vi "Build Evaluation String.vi"(6 "VI Path":path, 7 "Assert Scripting Configuration":T1={"Assert Name"="", "Comment"="", "Numeric Operation"="", "Type"=enum."Double Float", "String Operation"="", "DBL Comparison Value 1"=0.0, "DBL Comparison Value 2"=0.0, "I32 Comparison Value 1"=0, "I32 Comparison Value 2"=0, "Creator"="", "Creation Timestamp"=timestamp(0 s since 1904-01-01), "String Comparison Value"="", "Description"="", "Default Failure Action"=enum."None", "Boolean Comparison Value"=FALSE, "I8 Comparison Value 1"=0, "I8 Comparison Value 2"=0, "I16 Comparison Value 1"=0, "I16 Comparison Value 2"=0, "I64 Comparison Value 1"=0, "I64 Comparison Value 2"=0, "U8 Comparison Value 1"=0, "U8 Comparison Value 2"=0, "U16 Comparison Value 1"=0, "U16 Comparison Value 2"=0, "U32 Comparison Value 1"=0, "U32 Comparison Value 2"=0, "U64 Comparison Value 1"=0, "U64 Comparison Value 2"=0, "EXT Comparison Value 1"=0.0, "EXT Comparison Value 2"=0.0, "SGL Comparison Value 1"=0.0, "SGL Comparison Value 2"=0.0}, 8 "error in (no error)":errorcluster) -> (0 "error out":errorcluster, 2 "Evaluation String":string)   [LabVIEW 2016]
doc: "Builds up an evaluation string based on the input parameters specified and applies it to the new assert test vi."
uses:
  Assert Scripting Configuration.ctl
  <vilib>/Utility/Data Type/Type Definitions/Data Type.ctl
  <vilib>/Utility/error.llb/Error Cluster From Error Code.vi
  <vilib>/ErrorRing/Error Ring.xnode
  <vilib>/Utility/Data Type/NI_Data Type.lvlib
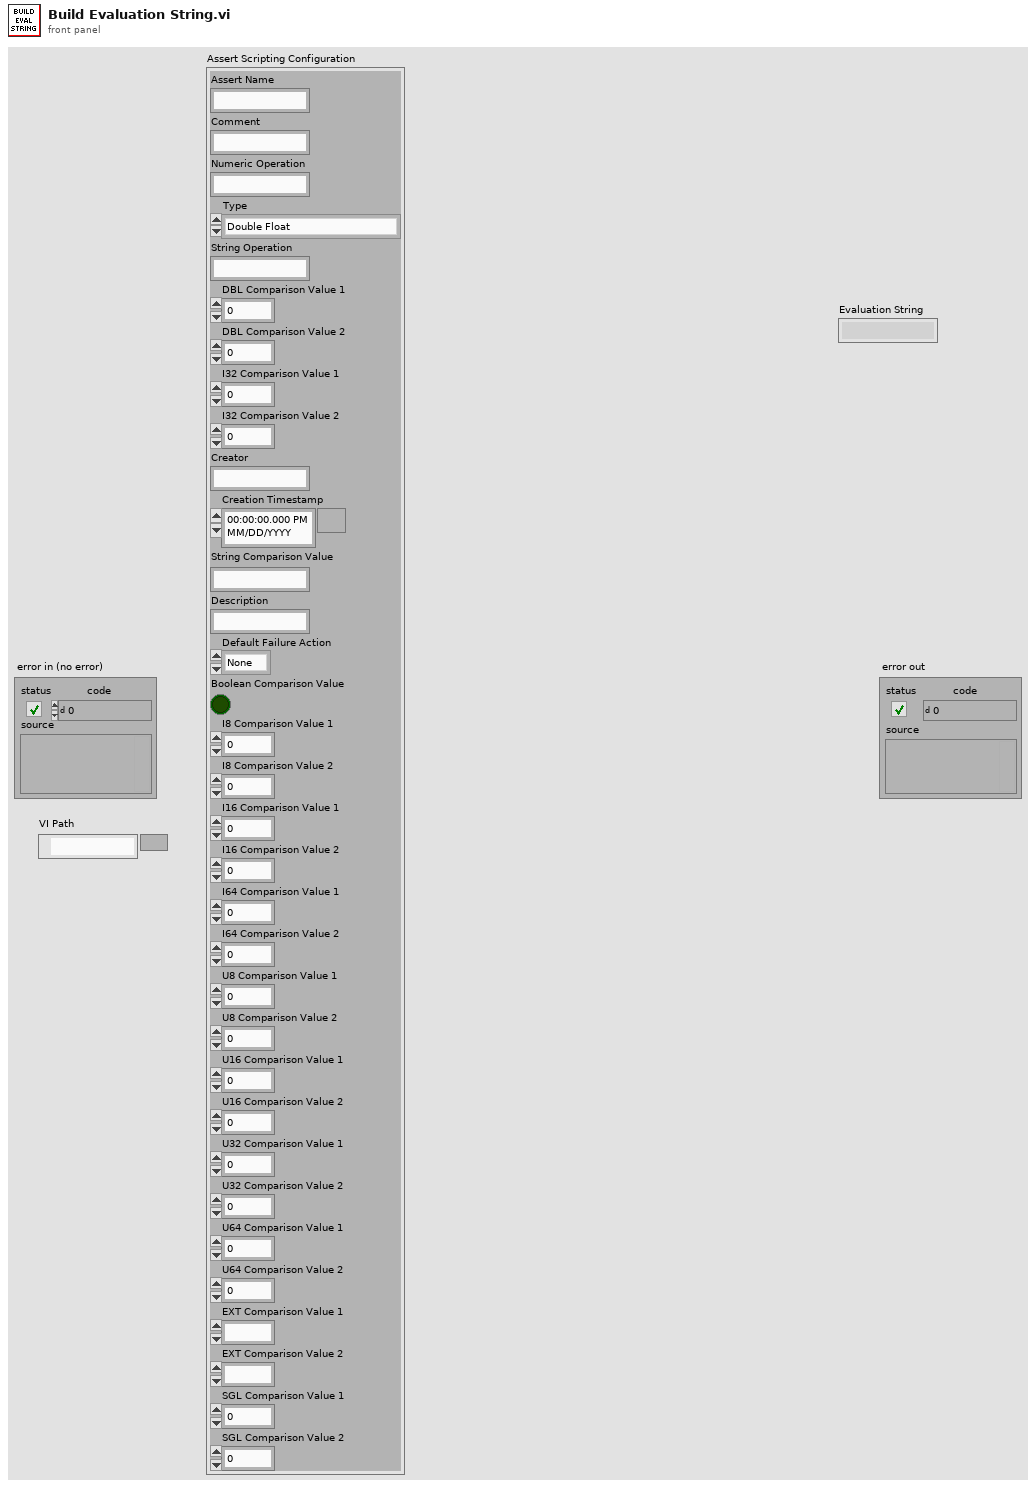
[diagram p1: front panel]
types:
  T1 = typedef "Assert Scripting Configuration.ctl" = cluster{"Assert Name":string, "Comment":string, "Numeric Operation":string, "Type":T2, "String Operation":string, "DBL Comparison Value 1":dbl, "DBL Comparison Value 2":dbl, "I32 Comparison Value 1":i32, "I32 Comparison Value 2":i32, "Creator":string, "Creation Timestamp":timestamp, "String Comparison Value":string, "Description":string, "Default Failure Action":enum16{"None", "Log To File", "Pause Execution", "Abort Execution"}, "Boolean Comparison Value":bool, "I8 Comparison Value 1":i8, "I8 Comparison Value 2":i8, "I16 Comparison Value 1":i16, "I16 Comparison Value 2":i16, "I64 Comparison Value 1":i64, "I64 Comparison Value 2":i64, "U8 Comparison Value 1":u8, "U8 Comparison Value 2":u8, "U16 Comparison Value 1":u16, "U16 Comparison Value 2":u16, "U32 Comparison Value 1":u32, "U32 Comparison Value 2":u32, "U64 Comparison Value 1":u64, "U64 Comparison Value 2":u64, "EXT Comparison Value 1":ext, "EXT Comparison Value 2":ext, "SGL Comparison Value 1":sgl, "SGL Comparison Value 2":sgl}
  T2 = typedef "NI_Data Type.lvlib/Data Type.ctl" = enum8{"Invalid Type", "Void", "I8", "I16", "I32", "I64", "U8", "U16", "U32", "U64", "Single Float", "Double Float", "Extended Float", "Single Complex", "Double Complex", "Extended Complex", "Enum U8", "Enum U16", "Enum U32", "Enum U64", "Single Float With Unit", "Double Float With Unit", "Extended Float With Unit", "Single Complex with Unit", "Double Complex with Unit", "Extended Complex with Unit", "Boolean", "String", "Path", "Picture", "Tag", "Array", "Cluster", "Variant", "LV Variant", "Waveform", "Timestamp", "Digital Waveform", "Digital Data", "ExpressData", "Refnum", "External Data", "VI", "Poly VI", "LabVIEW Class Instance", "Fixed Point"}
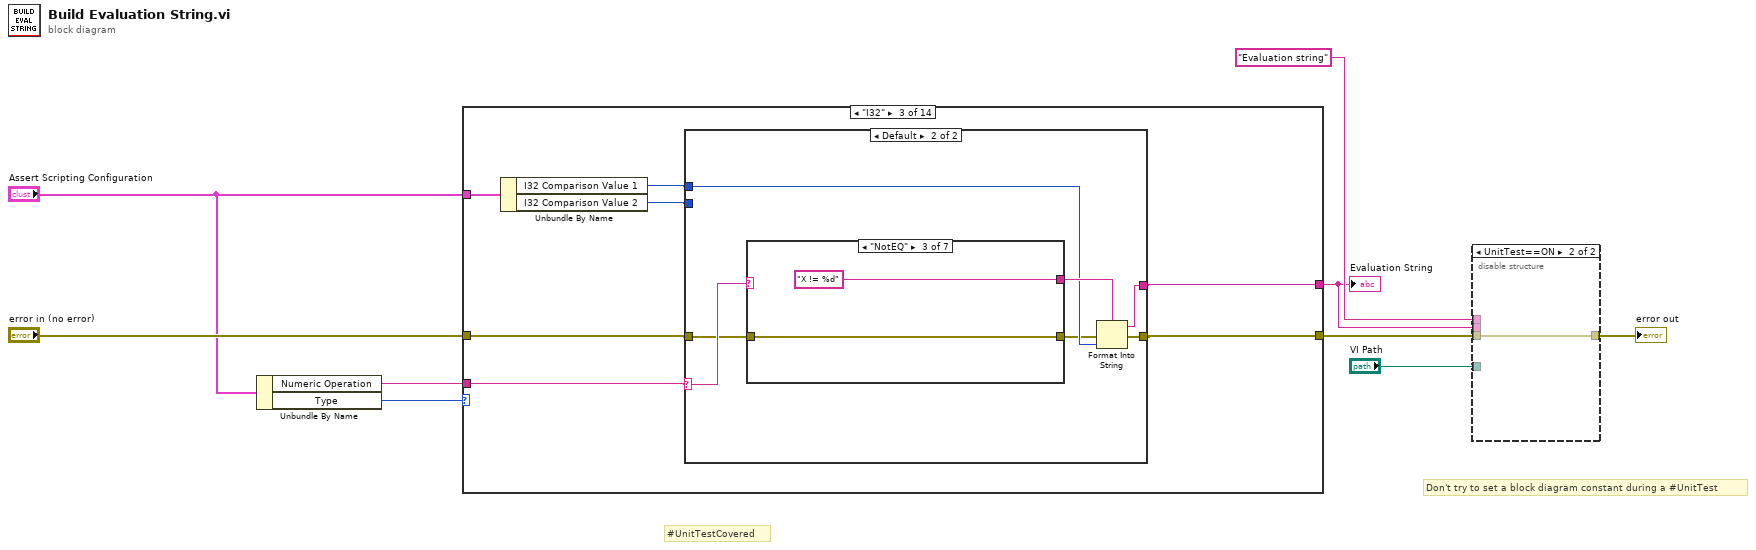
[diagram p0: block diagram]
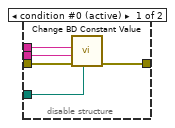
[diagram p2: hidden frame]
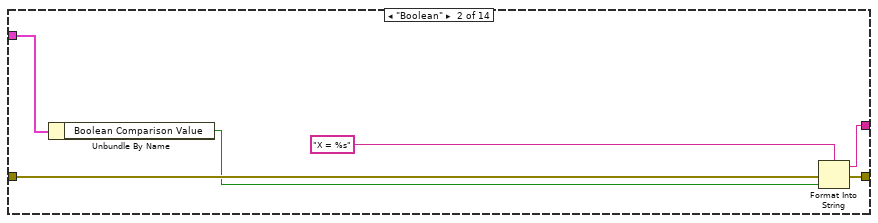
[diagram p4: hidden frame]
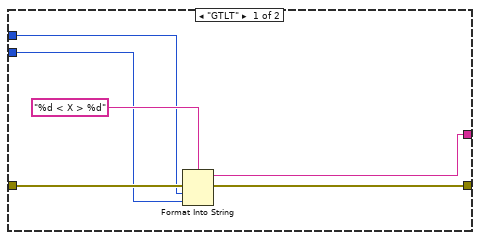
[diagram p5: hidden frame]
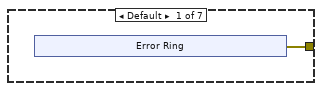
[diagram p6: hidden frame]
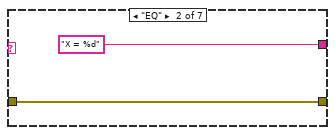
[diagram p7: hidden frame]
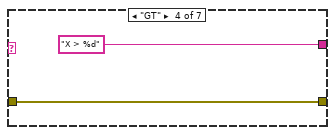
[diagram p8: hidden frame]
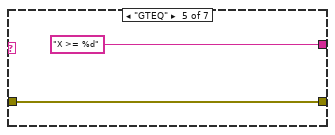
[diagram p9: hidden frame]
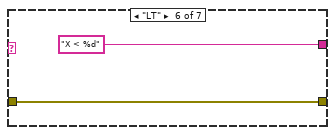
[diagram p10: hidden frame]
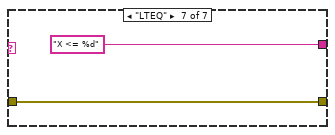
[diagram p11: hidden frame]
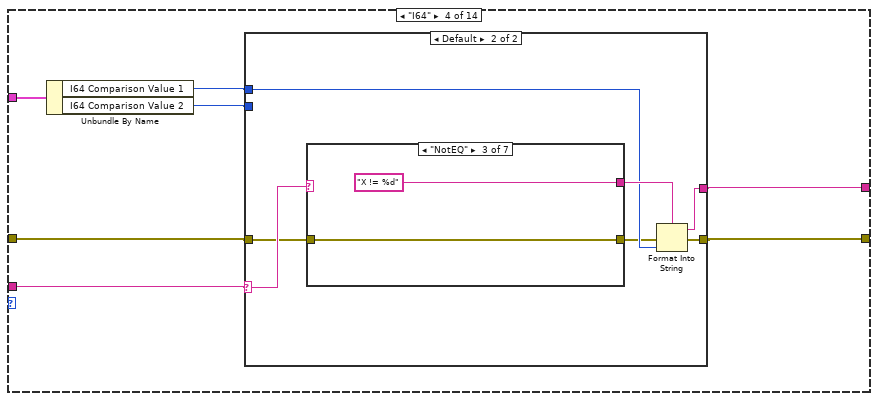
[diagram p12: hidden frame]
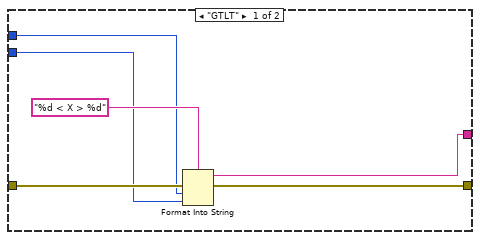
[diagram p13: hidden frame]
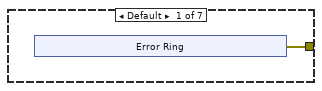
[diagram p14: hidden frame]
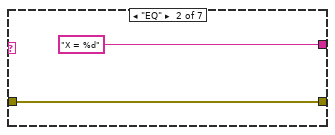
[diagram p15: hidden frame]
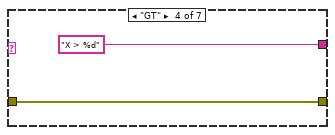
[diagram p16: hidden frame]
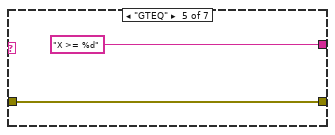
[diagram p17: hidden frame]
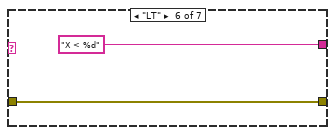
[diagram p18: hidden frame]
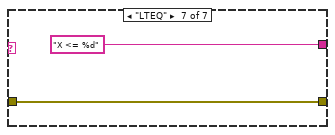
[diagram p19: hidden frame]
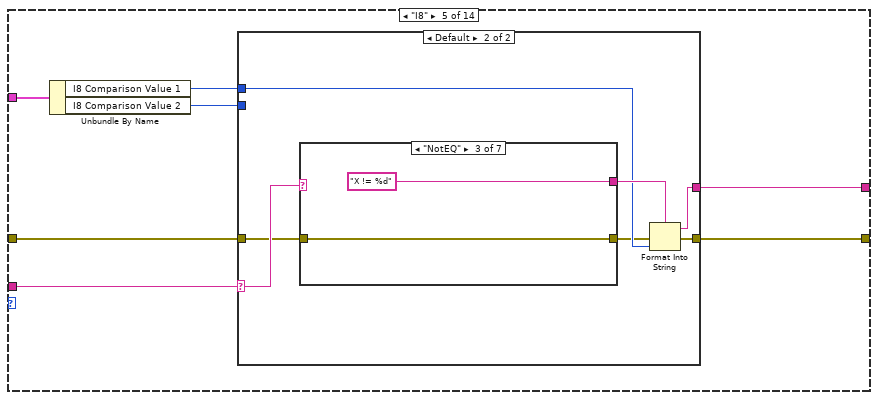
[diagram p20: hidden frame]
diagram:
  # "#UnitTestCovered"
  # "Don't try to set a block diagram constant during a #UnitTest"
  n1 = Unbundle By Name("Assert Scripting Configuration") -> ("Numeric Operation"=w7:string, "Type"=w8:T2)
  n2 = case shown="\"I32\"" w8 {
    tunnel: w7 -> [_ _ w22 w60 w98 w136 w174 w209 w250 w286 w323 w364 w403 _]
    tunnel: [_ w15 w18 w56 w94 w132 w170 w207 w246 w283 w321 w360 w402 w438] -> w5
    tunnel: "error in (no error)" -> [w10 w14 w21 w59 w97 w135 w173 w210 w249 w285 w324 w363 w401 w441]
    tunnel: [w10 w13 w17 w55 w93 w131 w169 w208 w245 w284 w322 w359 w400 w440] -> w4
    tunnel: "Assert Scripting Configuration" -> [_ w12 w23 w61 w99 w137 w175 w213 w251 w289 w327 w365 w399 w437]
    frame Default {
    }
    frame "Boolean" {
      n3 = Unbundle By Name(w12) -> ("Boolean Comparison Value"=w11:bool)
      n4 = Format Into String(format string="X = %s", error in=w14, w11) -> (resulting string=w15:string, error out=w13:errorcluster)  [unwired: 1 in]
    }
    frame "I32" {
      n5 = Unbundle By Name(w23) -> ("I32 Comparison Value 1"=w19:i32, "I32 Comparison Value 2"=w20:i32)
      n6 = case shown="Default" w22 {
        selector: w22 -> [_ w36]
        tunnel: [w28 w34] -> w18
        tunnel: w21 -> [w27 w31]
        tunnel: [w26 w33] -> w17
        tunnel: w19 -> [w25 w32]
        tunnel: w20 -> [w24 _]
        frame "GTLT" {
          n7 = Format Into String(format string="%d < X > %d", error in=w27, w25, w24) -> (resulting string=w28:string, error out=w26:errorcluster)  [unwired: 1 in]
        }
        frame Default {
          n8 = case shown="\"NotEQ\"" w36 {
            tunnel: [_ "X = %d" "X != %d" "X > %d" "X >= %d" "X < %d" "X <= %d"] -> w35
            tunnel: w31 -> [_ w43 w45 w47 w49 w51 w53]
            tunnel: [w37 w43 w45 w47 w49 w51 w53] -> w30
            frame Default {
              n9 = xnode "Error Ring"() -> ("error out"=w37:errorcluster)
            }
            frame "EQ" {
            }
            frame "NotEQ" {
            }
            frame "GT" {
            }
            frame "GTEQ" {
            }
            frame "LT" {
            }
            frame "LTEQ" {
            }
          }
          n10 = Format Into String(format string=w35, error in=w30, w32) -> (resulting string=w34:string, error out=w33:errorcluster)  [unwired: 1 in]
        }
      }
    }
    frame "I64" {
      n11 = Unbundle By Name(w61) -> ("I64 Comparison Value 1"=w57:i64, "I64 Comparison Value 2"=w58:i64)
      n12 = case shown="Default" w60 {
        selector: w60 -> [_ w74]
        tunnel: [w66 w72] -> w56
        tunnel: w59 -> [w65 w69]
        tunnel: [w64 w71] -> w55
        tunnel: w57 -> [w63 w70]
        tunnel: w58 -> [w62 _]
        frame "GTLT" {
          n13 = Format Into String(format string="%d < X > %d", error in=w65, w63, w62) -> (resulting string=w66:string, error out=w64:errorcluster)  [unwired: 1 in]
        }
        frame Default {
          n14 = case shown="\"NotEQ\"" w74 {
            tunnel: [_ "X = %d" "X != %d" "X > %d" "X >= %d" "X < %d" "X <= %d"] -> w73
            tunnel: w69 -> [_ w81 w83 w85 w87 w89 w91]
            tunnel: [w75 w81 w83 w85 w87 w89 w91] -> w68
            frame Default {
              n15 = xnode "Error Ring"() -> ("error out"=w75:errorcluster)
            }
            frame "EQ" {
            }
            frame "NotEQ" {
            }
            frame "GT" {
            }
            frame "GTEQ" {
            }
            frame "LT" {
            }
            frame "LTEQ" {
            }
          }
          n16 = Format Into String(format string=w73, error in=w68, w70) -> (resulting string=w72:string, error out=w71:errorcluster)  [unwired: 1 in]
        }
      }
    }
    frame "I8" {
      n17 = Unbundle By Name(w99) -> ("I8 Comparison Value 1"=w95:i8, "I8 Comparison Value 2"=w96:i8)
      n18 = case shown="Default" w98 {
        selector: w98 -> [_ w112]
        tunnel: [w104 w110] -> w94
        tunnel: w97 -> [w103 w107]
        tunnel: [w102 w109] -> w93
        tunnel: w95 -> [w101 w108]
        tunnel: w96 -> [w100 _]
        frame "GTLT" {
          n19 = Format Into String(format string="%d < X > %d", error in=w103, w101, w100) -> (resulting string=w104:string, error out=w102:errorcluster)  [unwired: 1 in]
        }
        frame Default {
          n20 = case shown="\"NotEQ\"" w112 {
            tunnel: [_ "X = %d" "X != %d" "X > %d" "X >= %d" "X < %d" "X <= %d"] -> w111
            tunnel: w107 -> [_ w119 w121 w123 w125 w127 w129]
            tunnel: [w113 w119 w121 w123 w125 w127 w129] -> w106
            frame Default {
              n21 = xnode "Error Ring"() -> ("error out"=w113:errorcluster)
            }
            frame "EQ" {
            }
            frame "NotEQ" {
            }
            frame "GT" {
            }
            frame "GTEQ" {
            }
            frame "LT" {
            }
            frame "LTEQ" {
            }
          }
          n22 = Format Into String(format string=w111, error in=w106, w108) -> (resulting string=w110:string, error out=w109:errorcluster)  [unwired: 1 in]
        }
      }
    }
    frame "I16" {
      n23 = Unbundle By Name(w137) -> ("I16 Comparison Value 1"=w133:i16, "I16 Comparison Value 2"=w134:i16)
      n24 = case shown="Default" w136 {
        selector: w136 -> [_ w150]
        tunnel: [w142 w148] -> w132
        tunnel: w135 -> [w141 w145]
        tunnel: [w140 w147] -> w131
        tunnel: w133 -> [w139 w146]
        tunnel: w134 -> [w138 _]
        frame "GTLT" {
          n25 = Format Into String(format string="%d < X > %d", error in=w141, w139, w138) -> (resulting string=w142:string, error out=w140:errorcluster)  [unwired: 1 in]
        }
        frame Default {
          n26 = case shown="\"NotEQ\"" w150 {
            tunnel: [_ "X = %d" "X != %d" "X > %d" "X >= %d" "X < %d" "X <= %d"] -> w149
            tunnel: w145 -> [_ w157 w159 w161 w163 w165 w167]
            tunnel: [w151 w157 w159 w161 w163 w165 w167] -> w144
            frame Default {
              n27 = xnode "Error Ring"() -> ("error out"=w151:errorcluster)
            }
            frame "EQ" {
            }
            frame "NotEQ" {
            }
            frame "GT" {
            }
            frame "GTEQ" {
            }
            frame "LT" {
            }
            frame "LTEQ" {
            }
          }
          n28 = Format Into String(format string=w149, error in=w144, w146) -> (resulting string=w148:string, error out=w147:errorcluster)  [unwired: 1 in]
        }
      }
    }
    frame "U8" {
      n29 = Unbundle By Name(w175) -> ("U8 Comparison Value 1"=w171:u8, "U8 Comparison Value 2"=w172:u8)
      n30 = case shown="Default" w174 {
        selector: w174 -> [_ w188]
        tunnel: [w180 w186] -> w170
        tunnel: w173 -> [w179 w183]
        tunnel: [w178 w185] -> w169
        tunnel: w171 -> [w177 w184]
        tunnel: w172 -> [w176 _]
        frame "GTLT" {
          n31 = Format Into String(format string="%d < X > %d", error in=w179, w177, w176) -> (resulting string=w180:string, error out=w178:errorcluster)  [unwired: 1 in]
        }
        frame Default {
          n32 = case shown="\"NotEQ\"" w188 {
            tunnel: [_ "X = %d" "X != %d" "X > %d" "X >= %d" "X < %d" "X <= %d"] -> w187
            tunnel: w183 -> [_ w195 w197 w199 w201 w203 w205]
            tunnel: [w189 w195 w197 w199 w201 w203 w205] -> w182
            frame Default {
              n33 = xnode "Error Ring"() -> ("error out"=w189:errorcluster)
            }
            frame "EQ" {
            }
            frame "NotEQ" {
            }
            frame "GT" {
            }
            frame "GTEQ" {
            }
            frame "LT" {
            }
            frame "LTEQ" {
            }
          }
          n34 = Format Into String(format string=w187, error in=w182, w184) -> (resulting string=w186:string, error out=w185:errorcluster)  [unwired: 1 in]
        }
      }
    }
    frame "U16" {
      n35 = Unbundle By Name(w213) -> ("U16 Comparison Value 1"=w212:u16, "U16 Comparison Value 2"=w211:u16)
      n36 = case shown="Default" w209 {
        selector: w209 -> [_ w226]
        tunnel: [w218 w224] -> w207
        tunnel: w210 -> [w217 w221]
        tunnel: [w216 w223] -> w208
        tunnel: w212 -> [w215 w222]
        tunnel: w211 -> [w214 _]
        frame "GTLT" {
          n37 = Format Into String(format string="%d < X > %d", error in=w217, w215, w214) -> (resulting string=w218:string, error out=w216:errorcluster)  [unwired: 1 in]
        }
        frame Default {
          n38 = case shown="\"NotEQ\"" w226 {
            tunnel: [_ "X = %d" "X != %d" "X > %d" "X >= %d" "X < %d" "X <= %d"] -> w225
            tunnel: w221 -> [_ w233 w235 w237 w239 w241 w243]
            tunnel: [w227 w233 w235 w237 w239 w241 w243] -> w220
            frame Default {
              n39 = xnode "Error Ring"() -> ("error out"=w227:errorcluster)
            }
            frame "EQ" {
            }
            frame "NotEQ" {
            }
            frame "GT" {
            }
            frame "GTEQ" {
            }
            frame "LT" {
            }
            frame "LTEQ" {
            }
          }
          n40 = Format Into String(format string=w225, error in=w220, w222) -> (resulting string=w224:string, error out=w223:errorcluster)  [unwired: 1 in]
        }
      }
    }
    frame "U32" {
      n41 = Unbundle By Name(w251) -> ("U32 Comparison Value 1"=w247:u32, "U32 Comparison Value 2"=w248:u32)
      n42 = case shown="Default" w250 {
        selector: w250 -> [_ w264]
        tunnel: [w256 w262] -> w246
        tunnel: w249 -> [w255 w259]
        tunnel: [w254 w261] -> w245
        tunnel: w247 -> [w253 w260]
        tunnel: w248 -> [w252 _]
        frame "GTLT" {
          n43 = Format Into String(format string="%d < X > %d", error in=w255, w253, w252) -> (resulting string=w256:string, error out=w254:errorcluster)  [unwired: 1 in]
        }
        frame Default {
          n44 = case shown="\"NotEQ\"" w264 {
            tunnel: [_ "X = %d" "X != %d" "X > %d" "X >= %d" "X < %d" "X <= %d"] -> w263
            tunnel: w259 -> [_ w271 w273 w275 w277 w279 w281]
            tunnel: [w265 w271 w273 w275 w277 w279 w281] -> w258
            frame Default {
              n45 = xnode "Error Ring"() -> ("error out"=w265:errorcluster)
            }
            frame "EQ" {
            }
            frame "NotEQ" {
            }
            frame "GT" {
            }
            frame "GTEQ" {
            }
            frame "LT" {
            }
            frame "LTEQ" {
            }
          }
          n46 = Format Into String(format string=w263, error in=w258, w260) -> (resulting string=w262:string, error out=w261:errorcluster)  [unwired: 1 in]
        }
      }
    }
    frame "U64" {
      n47 = Unbundle By Name(w289) -> ("U64 Comparison Value 1"=w288:u64, "U64 Comparison Value 2"=w287:u64)
      n48 = case shown="Default" w286 {
        selector: w286 -> [_ w302]
        tunnel: [w294 w300] -> w283
        tunnel: w285 -> [w293 w297]
        tunnel: [w292 w299] -> w284
        tunnel: w288 -> [w291 w298]
        tunnel: w287 -> [w290 _]
        frame "GTLT" {
          n49 = Format Into String(format string="%d < X > %d", error in=w293, w291, w290) -> (resulting string=w294:string, error out=w292:errorcluster)  [unwired: 1 in]
        }
        frame Default {
          n50 = case shown="\"NotEQ\"" w302 {
            tunnel: [_ "X = %d" "X != %d" "X > %d" "X >= %d" "X < %d" "X <= %d"] -> w301
            tunnel: w297 -> [_ w309 w311 w313 w315 w317 w319]
            tunnel: [w303 w309 w311 w313 w315 w317 w319] -> w296
            frame Default {
              n51 = xnode "Error Ring"() -> ("error out"=w303:errorcluster)
            }
            frame "EQ" {
            }
            frame "NotEQ" {
            }
            frame "GT" {
            }
            frame "GTEQ" {
            }
            frame "LT" {
            }
            frame "LTEQ" {
            }
          }
          n52 = Format Into String(format string=w301, error in=w296, w298) -> (resulting string=w300:string, error out=w299:errorcluster)  [unwired: 1 in]
        }
      }
    }
    frame "Double Float" {
      n53 = Unbundle By Name(w327) -> ("DBL Comparison Value 1"=w325:dbl, "DBL Comparison Value 2"=w326:dbl)
      n54 = case shown="\"GTLT\"" w323 {
        selector: w323 -> [_ w340]
        tunnel: [w332 w338] -> w321
        tunnel: w324 -> [w331 w335]
        tunnel: [w330 w337] -> w322
        tunnel: w325 -> [w329 w336]
        tunnel: w326 -> [w328 _]
        frame "GTLT" {
          n55 = Format Into String(format string="%f < X > %f", error in=w331, w329, w328) -> (resulting string=w332:string, error out=w330:errorcluster)  [unwired: 1 in]
        }
        frame Default {
          n56 = case shown="\"EQ\"" w340 {
            tunnel: [_ "X = %f" "X != %f" "X > %f" "X >= %f" "X < %f" "X <= %f"] -> w339
            tunnel: w335 -> [_ w347 w349 w351 w353 w355 w357]
            tunnel: [w341 w347 w349 w351 w353 w355 w357] -> w334
            frame Default {
              n57 = xnode "Error Ring"() -> ("error out"=w341:errorcluster)
            }
            frame "EQ" {
            }
            frame "NotEQ" {
            }
            frame "GT" {
            }
            frame "GTEQ" {
            }
            frame "LT" {
            }
            frame "LTEQ" {
            }
          }
          n58 = Format Into String(format string=w339, error in=w334, w336) -> (resulting string=w338:string, error out=w337:errorcluster)  [unwired: 1 in]
        }
      }
    }
    frame "Extended Float" {
      n59 = Unbundle By Name(w365) -> ("EXT Comparison Value 1"=w361:ext, "EXT Comparison Value 2"=w362:ext)
      n60 = case shown="\"GTLT\"" w364 {
        selector: w364 -> [_ w378]
        tunnel: [w370 w376] -> w360
        tunnel: w363 -> [w369 w373]
        tunnel: [w368 w375] -> w359
        tunnel: w361 -> [w367 w374]
        tunnel: w362 -> [w366 _]
        frame "GTLT" {
          n61 = Format Into String(format string="%f < X > %f", error in=w369, w367, w366) -> (resulting string=w370:string, error out=w368:errorcluster)  [unwired: 1 in]
        }
        frame Default {
          n62 = case shown="\"EQ\"" w378 {
            tunnel: [_ "X = %f" "X != %f" "X > %f" "X >= %f" "X < %f" "X <= %f"] -> w377
            tunnel: w373 -> [_ w385 w387 w389 w391 w393 w395]
            tunnel: [w379 w385 w387 w389 w391 w393 w395] -> w372
            frame Default {
              n63 = xnode "Error Ring"() -> ("error out"=w379:errorcluster)
            }
            frame "EQ" {
            }
            frame "NotEQ" {
            }
            frame "GT" {
            }
            frame "GTEQ" {
            }
            frame "LT" {
            }
            frame "LTEQ" {
            }
          }
          n64 = Format Into String(format string=w377, error in=w372, w374) -> (resulting string=w376:string, error out=w375:errorcluster)  [unwired: 1 in]
        }
      }
    }
    frame "Single Float" {
      n65 = Unbundle By Name(w399) -> ("SGL Comparison Value 1"=w398:sgl, "SGL Comparison Value 2"=w397:sgl)
      n66 = case shown="Default" w403 {
        selector: w403 -> [_ w416]
        tunnel: [w408 w414] -> w402
        tunnel: w401 -> [w407 w411]
        tunnel: [w406 w413] -> w400
        tunnel: w398 -> [w405 w412]
        tunnel: w397 -> [w404 _]
        frame "GTLT" {
          n67 = Format Into String(format string="%f < X > %f", error in=w407, w405, w404) -> (resulting string=w408:string, error out=w406:errorcluster)  [unwired: 1 in]
        }
        frame Default {
          n68 = case shown="Default" w416 {
            tunnel: [_ "X = %f" "X != %f" "X > %f" "X >= %f" "X < %f" "X <= %f"] -> w415
            tunnel: w411 -> [_ w423 w425 w427 w429 w431 w433]
            tunnel: [w417 w423 w425 w427 w429 w431 w433] -> w410
            frame Default {
              n69 = xnode "Error Ring"() -> ("error out"=w417:errorcluster)
            }
            frame "EQ" {
            }
            frame "NotEQ" {
            }
            frame "GT" {
            }
            frame "GTEQ" {
            }
            frame "LT" {
            }
            frame "LTEQ" {
            }
          }
          n70 = Format Into String(format string=w415, error in=w410, w412) -> (resulting string=w414:string, error out=w413:errorcluster)  [unwired: 1 in]
        }
      }
    }
    frame "String" {
      n71 = Unbundle By Name(w437) -> ("String Operation"=w436:string, "String Comparison Value"=w435:string)
      n72 = case shown="\"NotContain\"" w436 {
        tunnel: [_ "String = \"%s\"" "String != \"%s\"" "String should contain \"%s\"" "String should not contain \"%s\"" "String start with \"%s\"" "String end with \"%s\""] -> w439
        frame Default {
        }
        frame "EQ" {
        }
        frame "NotEQ" {
        }
        frame "Contains" {
        }
        frame "NotContain" {
        }
        frame "SW" {
        }
        frame "EW" {
        }
      }
      n73 = Format Into String(format string=w439, error in=w441, w435) -> (resulting string=w438:string, error out=w440:errorcluster)  [unwired: 1 in]
    }
  }
  "Evaluation String" <- w5
  n74 = disable-structure shown="UnitTest==ON" {
    disable-tunnel: "Evaluation string" ("Constant Name") -> [w452 _]
    disable-tunnel: w5 -> [w451 _]
    disable-tunnel: w4 -> [w450 w453]
    disable-tunnel: [w449 w453] -> w3
    disable-tunnel: "VI Path" -> [w448 _]
    frame condition #0 (active) {
      n75 = call "Change BD Constant Value.vi"("Assert VI Path"=w448, "error in (no error)"=w450, "Data Value"=w451, "Constant Name"=w452) -> ("error out"=w449:errorcluster)  [unwired: 7 in]
    }
    frame condition #1 {
    }
  }
  "error out" <- w3
